vi "自动回放.vi"() -> ()   [LabVIEW 2020]
uses:
  <vilib>/Analysis/2dsp.llb/Real FFT.vi
  <vilib>/Analysis/NI_AALPro.lvlib
  <vilib>/measure/NI_MABase.lvlib
panel:
  out "更换文件夹":bool
  out "波形图":waveform(dbl)(graph)
  out "此文件夹下文件数量":i32
  in  "此文件夹下所有文件":i32(listbox)
  in  "索引":i32
  in  "分段采样数":i32=2048 min=0 max=1000000
  in  "采样率(Hz)":dbl=32000.0 min=0.0 max=1000000.0
  out "回放信号时域波形图":waveform(dbl)(graph)
  out "回放信号频谱图":waveform(dbl)(graph)
  out "此回放文件的路径":path
  in  "回放文件夹":path
  in  "回放按钮":bool
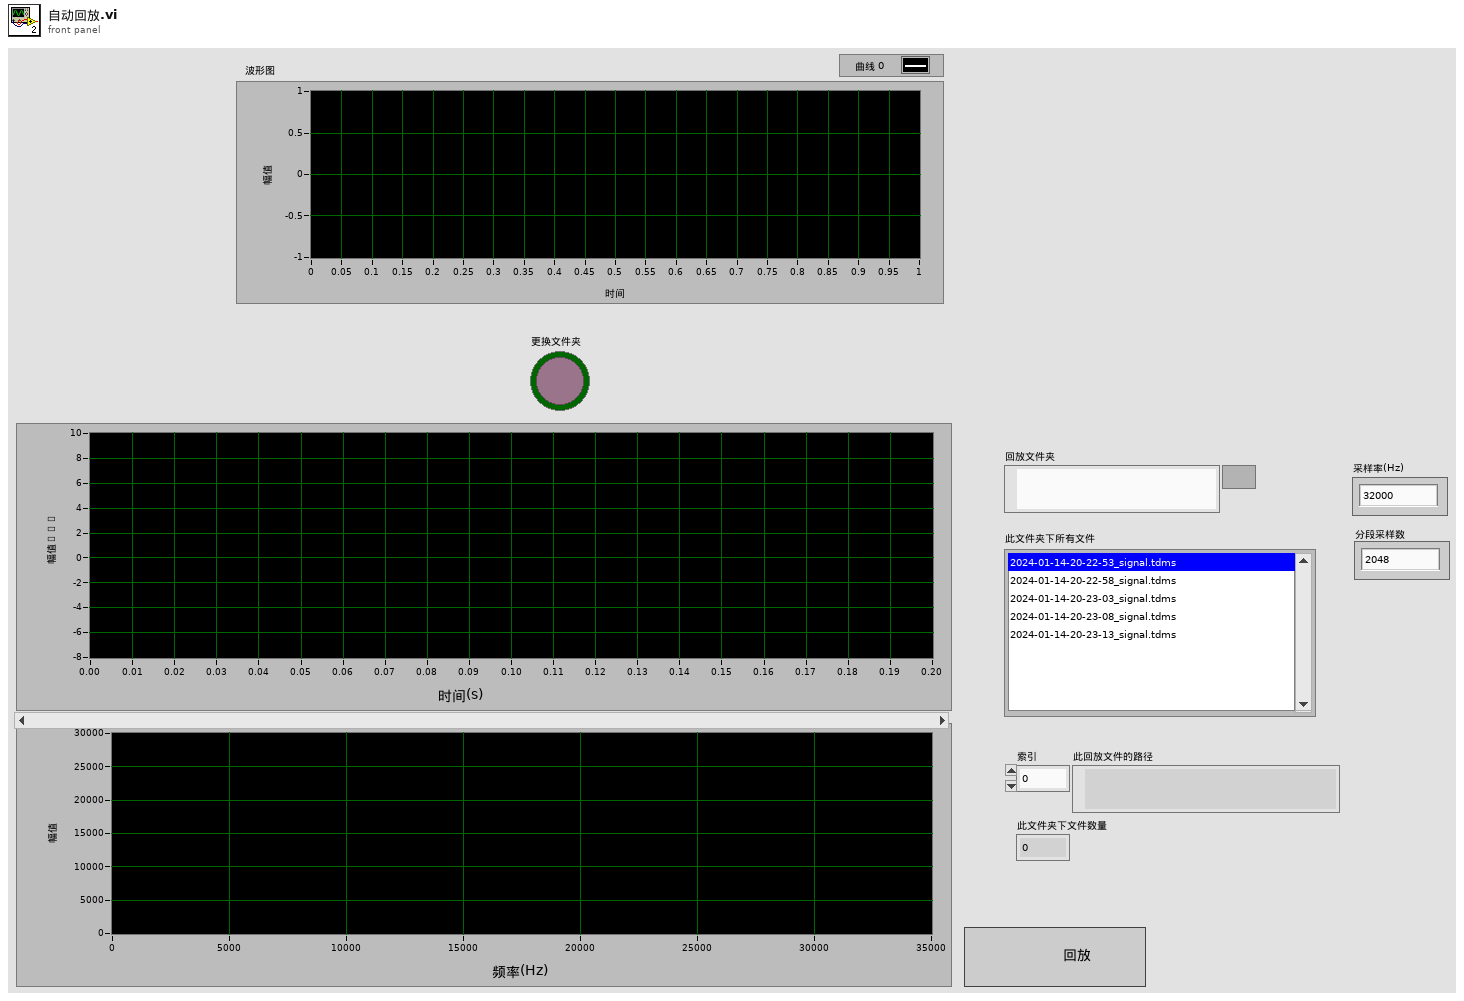
[diagram p1: front panel]
types:
  T1 = enum16{"open", "open or create", "create or replace", "create", "open (read-only)"}
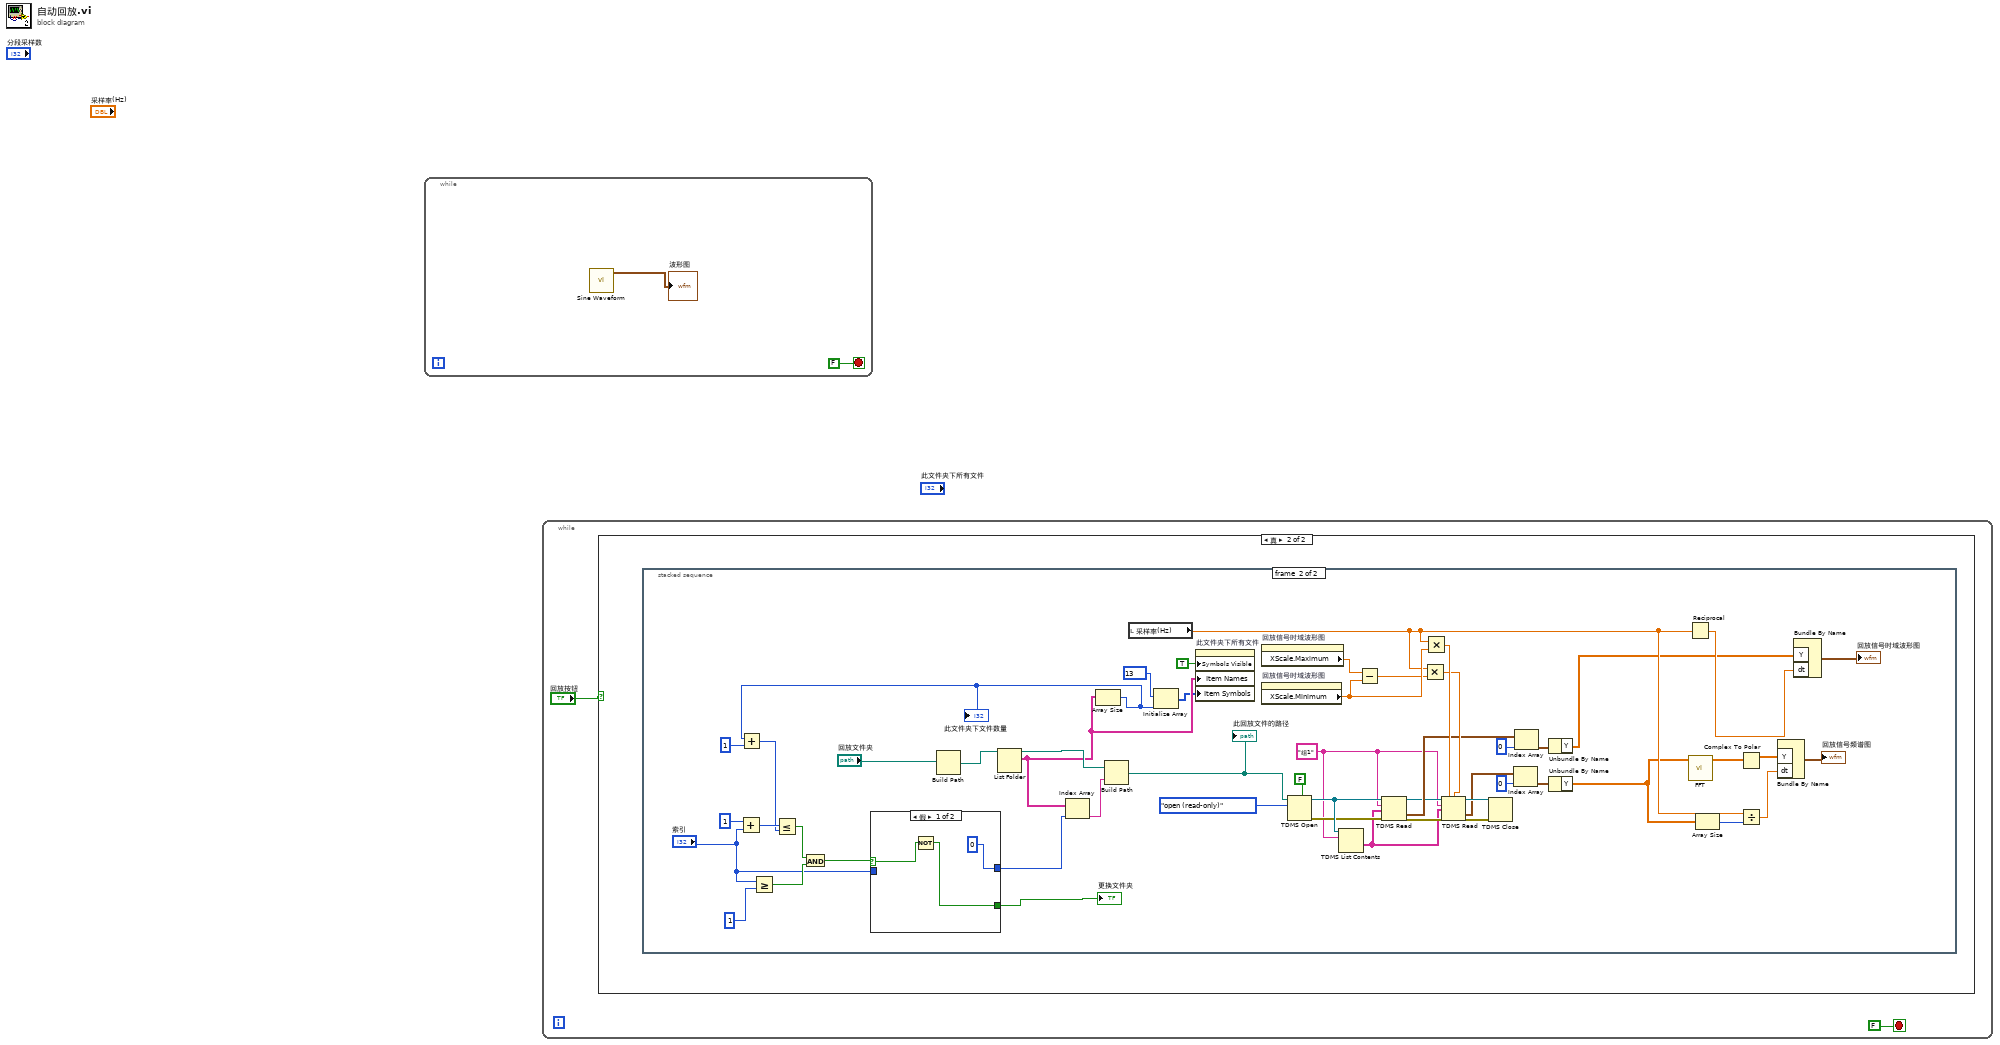
[diagram p0: block diagram]
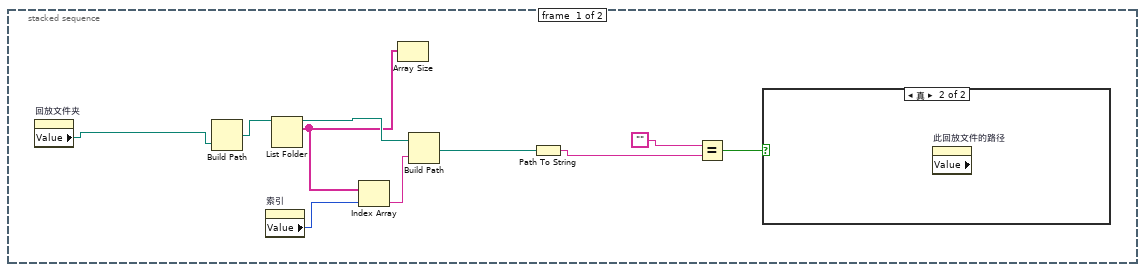
[diagram p3: hidden frame]
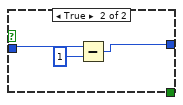
[diagram p5: hidden frame]
diagram:
  n1 = while {
    stop <- FALSE stop-if-true
    n2 = call <vilib>:"Sine Waveform.vi"() -> ("signal out"=→"波形图":waveform(dbl))  [unwired: 10 in, 1 out]
  }
  n3 = while {
    stop <- FALSE stop-if-true
    n4 = case shown="真" "回放按钮" {
      frame False {
      }
      frame True {
        n5 = stacked-sequence {
          frame #0 {
            n6 = property on="回放文件夹" class="Path"() -> ("Value"=w5:path)  [unwired: 2 in, 2 out]
            n7 = Build Path(name or relative path=w5) -> (appended path=w12:path)  [unwired: 1 in]
            n8 = property on="索引" class="DigNum (严格)"() -> ("Value"=w8:i32)  [unwired: 2 in, 2 out]
            n9 = List Folder(path=w12) -> (path out=w11:path, filenames=w9:string[])  [unwired: 3 in, 2 out]
            n10 = Index Array(array=w9, index=w8) -> (element=w10:string)
            n11 = Array Size(array=w9) -> ()  [unwired: 1 out]
            n12 = Build Path(base path=w11, name or relative path=w10) -> (appended path=w7:path)
            n13 = Path To String(path=w7) -> (string=w6:string)
            n14 = Equal?(x="", y=w6) -> (x = y?=w13:bool)
            n15 = case shown="真" w13 {
              frame False {
              }
              frame True {
                n16 = property on="此回放文件的路径" class="Path" props=["Value"]() -> ()  [unwired: 2 in, 3 out]
              }
            }
          }
          frame #1 {
            w39 = "组1" ("组名称输入")
            n17 = Add(x=1, y="索引") -> (x+y=w21:i32)
            n18 = Greater Or Equal?(x="索引", y=1) -> (x >= y?=w26:bool)
            n19 = Build Path(name or relative path="回放文件夹") -> (appended path=w51:path)  [unwired: 1 in]
            n20 = List Folder(path=w51) -> (path out=w50:path, filenames=w29:string[])  [unwired: 3 in, 2 out]
            n21 = Array Size(array=w29) -> (size(s)=w19:i32)
            "此文件夹下文件数量" <- w19
            n22 = Add(x=w19, y=1) -> (x+y=w17:i32)
            n23 = Less Or Equal?(x=w21, y=w17) -> (x <= y?=w20:bool)
            n24 = And(x=w20, y=w26) -> (x .and. y?=w25:bool)
            n25 = case shown="假" w25 {
              selector: w25 -> [w68 _]
              tunnel: [0 w70] -> w24
              tunnel: "索引" -> [_ w72]
              tunnel: [w67 _] -> w16
              frame False {
                n26 = Not(x=w68) -> (.not. x?=w67:bool)
              }
              frame True {
                n27 = Subtract(x=w72, y=1) -> (x-y=w70:i32)
              }
            }
            "更换文件夹" <- w16
            n28 = Index Array(array=w29, index=w24) -> (element=w33:string)
            n29 = Build Path(base path=w50, name or relative path=w33) -> (appended path=w34:path)
            "此回放文件的路径" <- w34
            n30 = local read "采样率(Hz)"() -> (w55:dbl)
            n31 = Initialize Array(13, w19) -> (w28:i32[])
            n32 = property on="此文件夹下所有文件" class="LstBox (严格)"("Symbols Visible"=TRUE ("显示项:显示符号"), "Item Names"=w29, "Item Symbols"=w28) -> ()  [unwired: 2 in, 2 out]
            n33 = property on="回放信号时域波形图" class="WFGraph (严格)"() -> ("XScale.Maximum"=w58:dbl)  [unwired: 2 in, 2 out]
            n34 = property on="回放信号时域波形图" class="WFGraph (严格)"() -> ("XScale.Minimum"=w57:dbl)  [unwired: 2 in, 2 out]
            n35 = TDMS Open(5:FALSE ("创建索引文件？(T)"), 10:T1."open (read-only)" ("操作(0:open)"), 11:w34) -> (0:w47:errorcluster, 3:w48:refnum<k34>)  [unwired: 4 in]
            n36 = TDMS List Contents(6:w39, 7:w48) -> (1:w38:string[])  [unwired: 1 in, 3 out]
            n37 = Subtract(x=w58, y=w57) -> (x-y=w56:dbl)
            n38 = TDMS Read(0:w48, 5:w39, 7:w38, 11:w47) -> (4:w43:refnum<k34>, 10:w45:waveform(dbl)[], 15:w42:errorcluster)  [unwired: 4 in, 3 out]
            n39 = Multiply(x=w55, y=w56) -> (x*y=w53:dbl)
            n40 = Multiply(x=w55, y=w57) -> (x*y=w59:dbl)
            n41 = TDMS Read(0:w43, 1:w59, 2:w53, 5:w39, 7:w38, 11:w42) -> (4:w41:refnum<k34>, 10:w36:waveform(dbl)[], 15:w40:errorcluster)  [unwired: 2 in, 3 out]
            n42 = TDMS Close(8:w40, 11:w41) -> ()  [unwired: 2 out]
            n43 = Index Array(array=w36, index=0 ("索引")) -> (element=w37:waveform(dbl))
            n44 = Index Array(array=w45, index=0 ("索引")) -> (element=w44:waveform(dbl))
            n45 = Unbundle By Name(w44) -> ("Y"=w15:dbl[])
            n46 = Unbundle By Name(w37) -> ("Y"=w54:dbl[])
            n47 = Reciprocal(x=w55) -> (1/x=w60:dbl)
            n48 = call-poly <vilib>:"FFT.vi"("X"=w54) -> ("FFT {X}"=w64:cdb[])  [unwired: 9 in, 1 out]
            n49 = Array Size(array=w54) -> (size(s)=w62:i32)
            n50 = Complex To Polar(r * e^(i*theta)=w64) -> (r=w65:dbl[])  [unwired: 1 out]
            n51 = Divide(x=w55, y=w62) -> (x/y=w66:dbl)
            n52 = Bundle By Name ("创建波形")("Y"=w65, "dt"=w66) -> (→"回放信号频谱图":waveform(dbl))  [unwired: 1 in]
            n53 = Bundle By Name("Y"=w15, "dt"=w60) -> (→"回放信号时域波形图":waveform(dbl))  [unwired: 1 in]
          }
        }
      }
    }
  }
